vi "ForceGraph1D.vi"(8 "number":dbl, 9 "Setpoint":dbl, 10 "k":dbl, 11 "Function":i32) -> (1 "force":dbl)   [LabVIEW 2023]
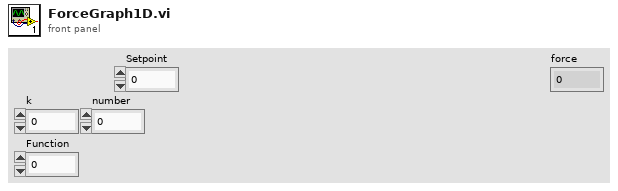
[diagram p1: front panel]
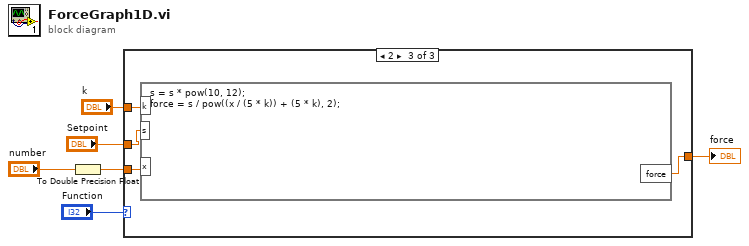
[diagram p0: block diagram]
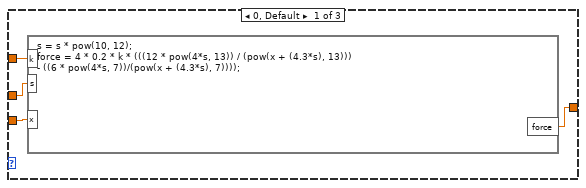
[diagram p2: hidden frame]
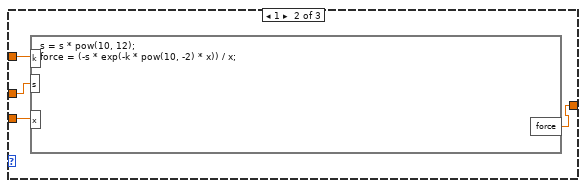
[diagram p3: hidden frame]
diagram:
  n1 = To Double Precision Float(number="number") -> (double precision float=w4:dbl)
  n2 = case shown="2" "Function" {
    tunnel: [w9 w14 w18] -> w2
    tunnel: w4 -> [w10 w13 w17]
    tunnel: "Setpoint" -> [w7 w12 w16]
    tunnel: "k" -> [w8 w11 w15]
    frame 0, Default {
      n3 = formula code="s = s * pow(10, 12);\nforce = 4 * 0.2 * k * (((12 * pow(4*s, 13)) / (pow(x + (4.3*s), 13))) \n- ((6 * pow(4*s, 7))/(pow(x + (4.3*s), 7))));"("x"=w10, "s"=w7, "k"=w8) -> ("force"=w9:dbl)
    }
    frame 1 {
      n4 = formula code="s = s * pow(10, 12);\nforce = (-s * exp(-k * pow(10, -2) * x)) / x;"("x"=w13, "s"=w12, "k"=w11) -> ("force"=w14:dbl)
    }
    frame 2 {
      n5 = formula code="s = s * pow(10, 12);\nforce = s / pow((x / (5 * k)) + (5 * k), 2);"("x"=w17, "s"=w16, "k"=w15) -> ("force"=w18:dbl)
    }
  }
  "force" <- w2
